vi "Stage_position_ae.vi"(8 "Status In":bool, 9 "Position In":dbl[](array[numeric]), 10 "StageID":string, 11 "Enum":enum16{"WRITE", "READ", "HOME", "SAVE HOME"}(ring)) -> (0 "Status Out":bool, 1 "Position Out":dbl[](array[numeric]))   [LabVIEW 2014]
panel:
  in  "Stage Home Positions":T1
  in  "Stage Status":T2
  in  "Stage Positions":T1
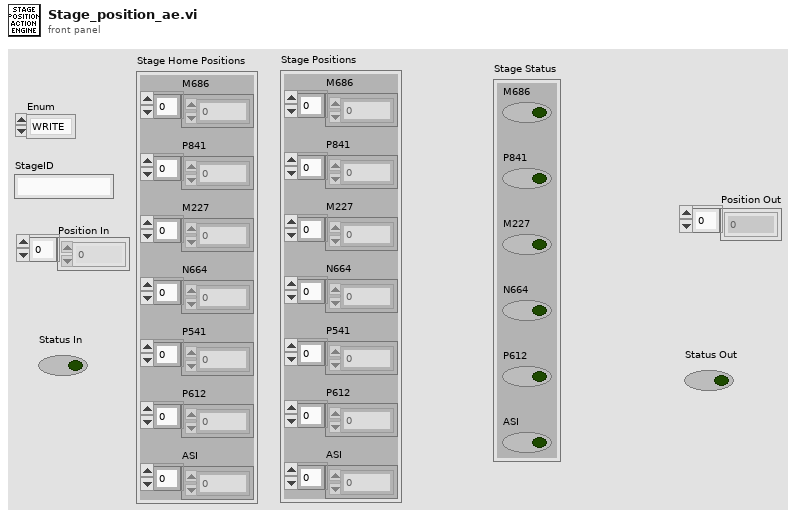
[diagram p1: front panel]
types:
  T1 = cluster{"M686":dbl[], "P841":dbl[], "M227":dbl[], "N664":dbl[], "P612":dbl[], "ASI":dbl[], "P541":dbl[]}
  T2 = cluster{"M686":bool, "P841":bool, "M227":bool, "N664":bool, "P612":bool, "ASI":bool}
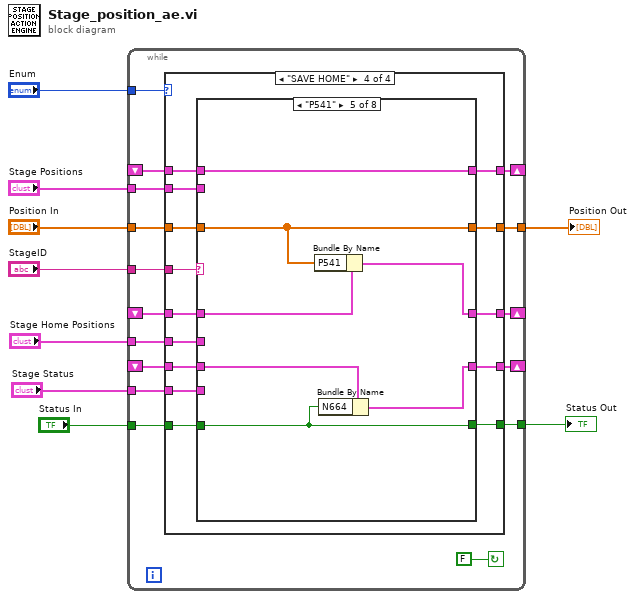
[diagram p0: block diagram]
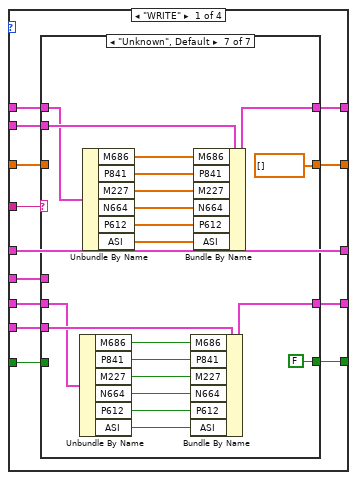
[diagram p2: hidden frame]
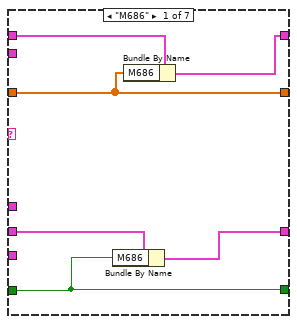
[diagram p3: hidden frame]
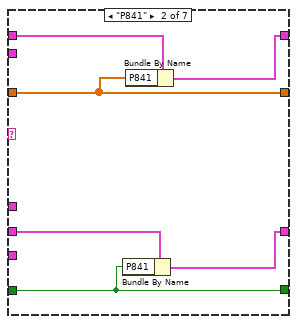
[diagram p4: hidden frame]
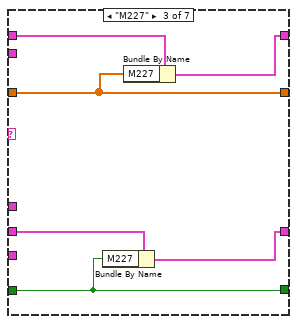
[diagram p5: hidden frame]
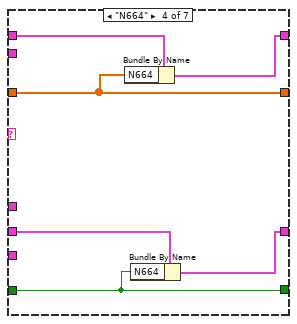
[diagram p6: hidden frame]
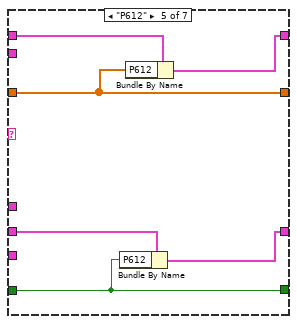
[diagram p7: hidden frame]
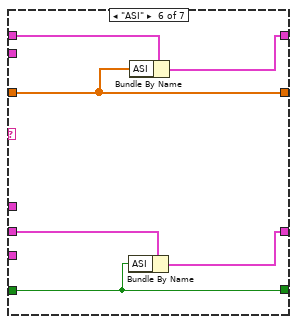
[diagram p8: hidden frame]
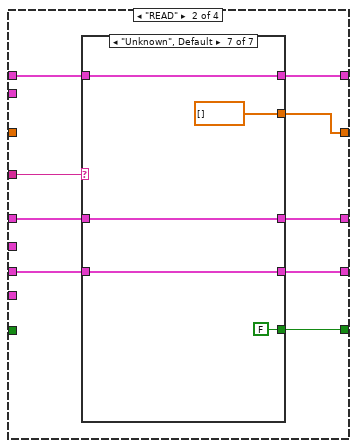
[diagram p9: hidden frame]
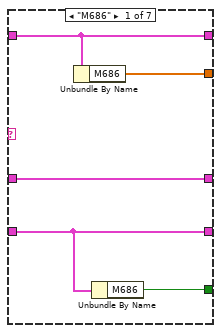
[diagram p10: hidden frame]
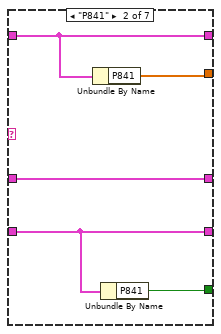
[diagram p11: hidden frame]
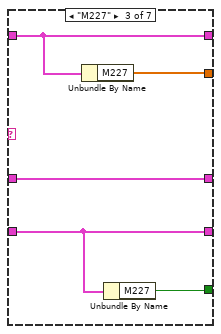
[diagram p12: hidden frame]
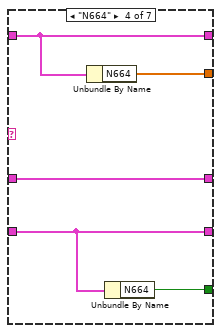
[diagram p13: hidden frame]
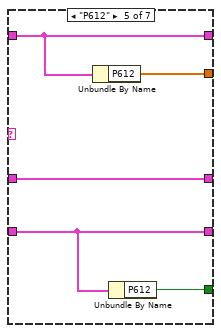
[diagram p14: hidden frame]
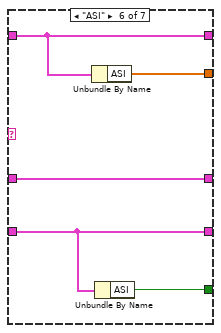
[diagram p15: hidden frame]
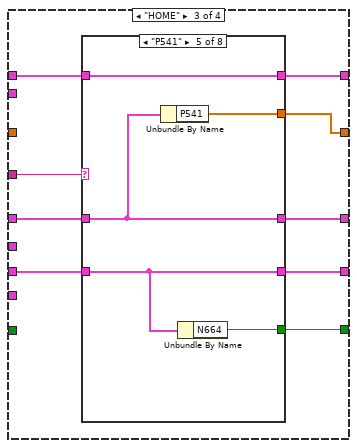
[diagram p16: hidden frame]
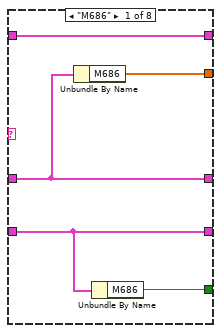
[diagram p17: hidden frame]
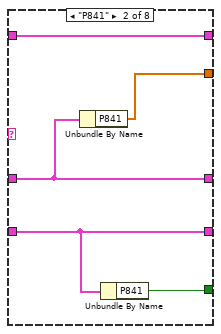
[diagram p18: hidden frame]
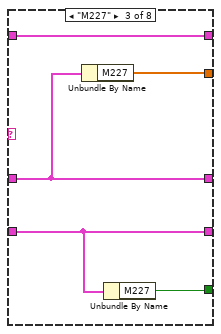
[diagram p19: hidden frame]
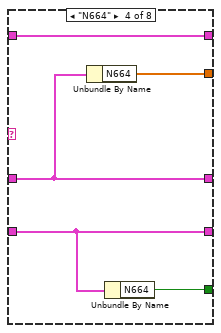
[diagram p20: hidden frame]
diagram:
  n1 = while {
    tunnel: "StageID" -> [w21]
    tunnel: "Enum" -> [w24]
    shift-right: [w23] -> _
    shift-left: _ -> [w22]
    tunnel: "Stage Positions" -> [w20]
    tunnel: "Position In" -> [w19]
    tunnel: [w18] -> w5
    shift-right: [w16] -> _
    shift-left: _ -> [w15]
    tunnel: "Stage Status" -> [w17]
    tunnel: [w14] -> w3
    tunnel: "Status In" -> [w13]
    shift-right: [w11] -> _
    shift-left: _ -> [w12]
    tunnel: "Stage Home Positions" -> [w10]
    stop <- FALSE continue-if-true
    n2 = case shown="\"SAVE HOME\"" w24 {
      tunnel: [w38 w103 w147 w201] -> w23
      tunnel: w22 -> [w33 w101 w145 w196]
      tunnel: w21 -> [w37 w102 w146 w200]
      tunnel: w20 -> [w36 _ _ w199]
      tunnel: w19 -> [w35 _ _ w198]
      tunnel: [w34 w100 w144 w197] -> w18
      tunnel: w17 -> [w32 _ _ w195]
      tunnel: [w31 w99 w143 w194] -> w16
      tunnel: w15 -> [w30 w98 w142 w193]
      tunnel: [w28 w97 w141 w191] -> w14
      tunnel: w13 -> [w29 _ _ w192]
      tunnel: w12 -> [w27 w96 w140 w190]
      tunnel: [w27 w95 w139 w189] -> w11
      tunnel: w10 -> [w26 _ _ w188]
      frame "WRITE" {
        n3 = case shown="\"Unknown\", Default" w37 {
          tunnel: [w44 w50 w56 w62 w68 w74 w93] -> w38
          tunnel: w36 -> [_ _ _ _ _ _ w94]
          tunnel: w35 -> [w43 w49 w55 w61 w67 w73 _]
          tunnel: [w43 w49 w55 w61 w67 w73 dbl[] [] ("VISA In")] -> w34
          tunnel: w33 -> [w42 w48 w54 w60 w66 w72 w92]
          tunnel: w32 -> [_ _ _ _ _ _ w81]
          tunnel: [w40 w46 w52 w57 w63 w70 w80] -> w31
          tunnel: w30 -> [w41 w47 w53 w58 w64 w71 w79]
          tunnel: w29 -> [w39 w45 w51 w59 w65 w69 _]
          tunnel: [w39 w45 w51 w59 w65 w69 FALSE ("Status In")] -> w28
          tunnel: w26 -> [_ _ _ _ _ _ _]
          frame "M686" {
            n4 = Bundle By Name(cluster=w41, "M686"=w39) -> (w40:T2)
            n5 = Bundle By Name(cluster=w42, "M686"=w43) -> (w44:T1)
          }
          frame "P841" {
            n6 = Bundle By Name(cluster=w47, "P841"=w45) -> (w46:T2)
            n7 = Bundle By Name(cluster=w48, "P841"=w49) -> (w50:T1)
          }
          frame "M227" {
            n8 = Bundle By Name(cluster=w53, "M227"=w51) -> (w52:T2)
            n9 = Bundle By Name(cluster=w54, "M227"=w55) -> (w56:T1)
          }
          frame "N664" {
            n10 = Bundle By Name(cluster=w60, "N664"=w61) -> (w62:T1)
            n11 = Bundle By Name(cluster=w58, "N664"=w59) -> (w57:T2)
          }
          frame "P612" {
            n12 = Bundle By Name(cluster=w64, "P612"=w65) -> (w63:T2)
            n13 = Bundle By Name(cluster=w66, "P612"=w67) -> (w68:T1)
          }
          frame "ASI" {
            n14 = Bundle By Name(cluster=w71, "ASI"=w69) -> (w70:T2)
            n15 = Bundle By Name(cluster=w72, "ASI"=w73) -> (w74:T1)
          }
          frame "Unknown", Default {
            n16 = Unbundle By Name(w79) -> ("M686"=w78:bool, "P841"=w77:bool, "M227"=w76:bool, "N664"=w82:bool, "P612"=w83:bool, "ASI"=w84:bool)
            n17 = Unbundle By Name(w92) -> ("M686"=w91:dbl[], "P841"=w90:dbl[], "M227"=w89:dbl[], "N664"=w88:dbl[], "P612"=w87:dbl[], "ASI"=w86:dbl[])
            n18 = Bundle By Name(cluster=w81, "M686"=w78, "P841"=w77, "M227"=w76, "N664"=w82, "P612"=w83, "ASI"=w84) -> (w80:T2)
            n19 = Bundle By Name(cluster=w94, "M686"=w91, "P841"=w90, "M227"=w89, "N664"=w88, "P612"=w87, "ASI"=w86) -> (w93:T1)
          }
        }
      }
      frame "READ" {
        n20 = case shown="\"Unknown\", Default" w102 {
          tunnel: [w108 w113 w118 w123 w128 w133 w138] -> w103
          tunnel: w101 -> [w108 w113 w118 w123 w128 w133 w138]
          tunnel: [w107 w112 w117 w122 w127 w132 dbl[] [] ("ASI_handle")] -> w100
          tunnel: [w106 w111 w116 w121 w126 w131 w136] -> w99
          tunnel: w98 -> [w106 w111 w116 w121 w126 w131 w136]
          tunnel: [w105 w110 w115 w120 w125 w130 FALSE ("ASI")] -> w97
          tunnel: w96 -> [w104 w109 w114 w119 w124 w129 w134]
          tunnel: [w104 w109 w114 w119 w124 w129 w134] -> w95
          frame "M686" {
            n21 = Unbundle By Name(w108) -> ("M686"=w107:dbl[])
            n22 = Unbundle By Name(w106) -> ("M686"=w105:bool)
          }
          frame "P841" {
            n23 = Unbundle By Name(w113) -> ("P841"=w112:dbl[])
            n24 = Unbundle By Name(w111) -> ("P841"=w110:bool)
          }
          frame "M227" {
            n25 = Unbundle By Name(w118) -> ("M227"=w117:dbl[])
            n26 = Unbundle By Name(w116) -> ("M227"=w115:bool)
          }
          frame "N664" {
            n27 = Unbundle By Name(w123) -> ("N664"=w122:dbl[])
            n28 = Unbundle By Name(w121) -> ("N664"=w120:bool)
          }
          frame "P612" {
            n29 = Unbundle By Name(w128) -> ("P612"=w127:dbl[])
            n30 = Unbundle By Name(w126) -> ("P612"=w125:bool)
          }
          frame "ASI" {
            n31 = Unbundle By Name(w133) -> ("ASI"=w132:dbl[])
            n32 = Unbundle By Name(w131) -> ("ASI"=w130:bool)
          }
          frame "Unknown", Default {
          }
        }
      }
      frame "HOME" {
        n33 = case shown="\"P541\"" w146 {
          tunnel: [w152 w157 w162 w167 w172 w177 w182 w187] -> w147
          tunnel: w145 -> [w152 w157 w162 w167 w172 w177 w182 w187]
          tunnel: [w151 w153 w161 w166 w171 w176 w181 dbl[] [] ("ASI_handle")] -> w144
          tunnel: [w150 w156 w160 w165 w170 w175 w180 w185] -> w143
          tunnel: w142 -> [w150 w156 w160 w165 w170 w175 w180 w185]
          tunnel: [w149 w155 w159 w164 w169 w174 w179 FALSE ("ASI")] -> w141
          tunnel: w140 -> [w148 w154 w158 w163 w168 w173 w178 w183]
          tunnel: [w148 w154 w158 w163 w168 w173 w178 w183] -> w139
          frame "M686" {
            n34 = Unbundle By Name(w148) -> ("M686"=w151:dbl[])
            n35 = Unbundle By Name(w150) -> ("M686"=w149:bool)
          }
          frame "P841" {
            n36 = Unbundle By Name(w154) -> ("P841"=w153:dbl[])
            n37 = Unbundle By Name(w156) -> ("P841"=w155:bool)
          }
          frame "M227" {
            n38 = Unbundle By Name(w158) -> ("M227"=w161:dbl[])
            n39 = Unbundle By Name(w160) -> ("M227"=w159:bool)
          }
          frame "N664" {
            n40 = Unbundle By Name(w163) -> ("N664"=w166:dbl[])
            n41 = Unbundle By Name(w165) -> ("N664"=w164:bool)
          }
          frame "P541" {
            n42 = Unbundle By Name(w168) -> ("P541"=w171:dbl[])
            n43 = Unbundle By Name(w170) -> ("N664"=w169:bool)
          }
          frame "P612" {
            n44 = Unbundle By Name(w173) -> ("P612"=w176:dbl[])
            n45 = Unbundle By Name(w175) -> ("P612"=w174:bool)
          }
          frame "ASI" {
            n46 = Unbundle By Name(w178) -> ("ASI"=w181:dbl[])
            n47 = Unbundle By Name(w180) -> ("ASI"=w179:bool)
          }
          frame "Unknown", Default {
          }
        }
      }
      frame "SAVE HOME" {
        n48 = case shown="\"P541\"" w200 {
          tunnel: [w204 w212 w218 w225 w232 w239 w246 w253] -> w201
          tunnel: w199 -> [_ _ _ _ _ _ _ _]
          tunnel: w198 -> [w208 w209 w222 w229 w236 w243 w250 _]
          tunnel: [w208 w209 w222 w229 w236 w243 w250 dbl[] [] ("VISA In")] -> w197
          tunnel: w196 -> [w204 w212 w218 w225 w232 w239 w246 w253]
          tunnel: w195 -> [_ _ _ _ _ _ _ w261]
          tunnel: [w206 w214 w220 w226 w233 w240 w248 w260] -> w194
          tunnel: w193 -> [w207 w215 w221 w227 w234 w241 w249 w259]
          tunnel: w192 -> [w205 w213 w219 w228 w235 w242 w247 _]
          tunnel: [w205 w213 w219 w228 w235 w242 w247 FALSE ("Status In")] -> w191
          tunnel: w190 -> [w203 w211 w217 w224 w231 w238 w245 w252]
          tunnel: [w202 w210 w216 w223 w230 w237 w244 w254] -> w189
          tunnel: w188 -> [_ _ _ _ _ _ _ w251]
          frame "M686" {
            n49 = Bundle By Name(cluster=w207, "M686"=w205) -> (w206:T2)
            n50 = Bundle By Name(cluster=w203, "M686"=w208) -> (w202:T1)
          }
          frame "P841" {
            n51 = Bundle By Name(cluster=w211, "P841"=w209) -> (w210:T1)
            n52 = Bundle By Name(cluster=w215, "P841"=w213) -> (w214:T2)
          }
          frame "M227" {
            n53 = Bundle By Name(cluster=w221, "M227"=w219) -> (w220:T2)
            n54 = Bundle By Name(cluster=w217, "M227"=w222) -> (w216:T1)
          }
          frame "N664" {
            n55 = Bundle By Name(cluster=w224, "N664"=w229) -> (w223:T1)
            n56 = Bundle By Name(cluster=w227, "N664"=w228) -> (w226:T2)
          }
          frame "P541" {
            n57 = Bundle By Name(cluster=w231, "P541"=w236) -> (w230:T1)
            n58 = Bundle By Name(cluster=w234, "N664"=w235) -> (w233:T2)
          }
          frame "P612" {
            n59 = Bundle By Name(cluster=w241, "P612"=w242) -> (w240:T2)
            n60 = Bundle By Name(cluster=w238, "P612"=w243) -> (w237:T1)
          }
          frame "ASI" {
            n61 = Bundle By Name(cluster=w249, "ASI"=w247) -> (w248:T2)
            n62 = Bundle By Name(cluster=w245, "ASI"=w250) -> (w244:T1)
          }
          frame "Unknown", Default {
            n63 = Unbundle By Name(w259) -> ("M686"=w258:bool, "P841"=w257:bool, "M227"=w256:bool, "N664"=w262:bool, "P612"=w263:bool, "ASI"=w264:bool)
            n64 = Unbundle By Name(w252) -> ("M686"=w271:dbl[], "P841"=w270:dbl[], "M227"=w269:dbl[], "N664"=w268:dbl[], "P612"=w267:dbl[], "ASI"=w266:dbl[])
            n65 = Bundle By Name(cluster=w261, "M686"=w258, "P841"=w257, "M227"=w256, "N664"=w262, "P612"=w263, "ASI"=w264) -> (w260:T2)
            n66 = Bundle By Name(cluster=w251, "M686"=w271, "P841"=w270, "M227"=w269, "N664"=w268, "P612"=w267, "ASI"=w266) -> (w254:T1)
          }
        }
      }
    }
  }
  "Position Out" <- w5
  "Status Out" <- w3
